vi "Previous Song.vi"(0 "reference in":refnum<class "MusicPlayer.lvclass">, 11 "Error In":errorcluster) -> (4 "reference out":refnum<class "MusicPlayer.lvclass">, 15 "Error Out":errorcluster)   [LabVIEW 2022 SP3, in "MusicPlayer.lvclass"]
uses:
  MusicPlayer.lvclass
  MusicPlayer.lvclass/MusicPlayer.ctl
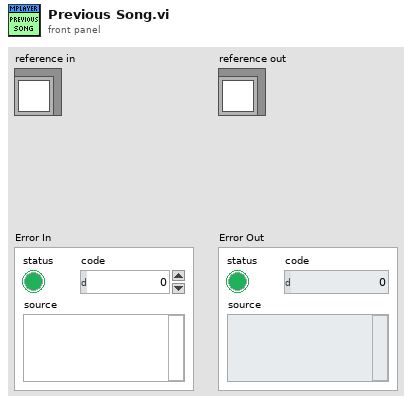
[diagram p1: front panel]
types:
  T1 = typedef "MusicPlayer.lvclass/ObjectAttributes.ctl" = cluster{"MediaPlayer":refnum<k7>, "Playlist":path[], "Index":u32}
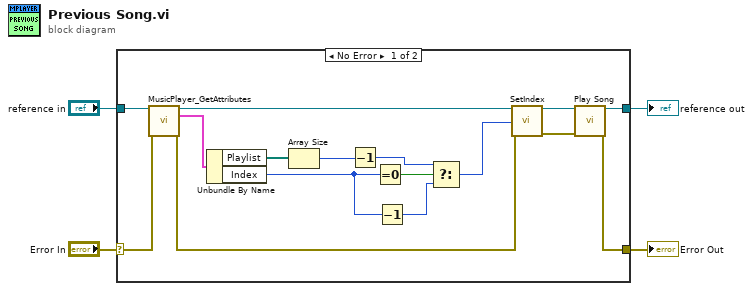
[diagram p0: block diagram]
diagram:
  n1 = case shown="No Error" "Error In" {
    selector: "Error In" -> [w20 w22]
    tunnel: [w8 w22] -> w3
    tunnel: [w6 w21] -> w1
    tunnel: "reference in" -> [w17 w21]
    frame No Error {
      n2 = call "MusicPlayer_GetAttributes.vi"("reference in"=w17, "error in (no error)"=w20) -> ("reference out"=w9:refnum<class "MusicPlayer.lvclass">, "Data"=w19:T1, "error out"=w18:errorcluster)  [unwired: 10 in, 1 out]
      n3 = Unbundle By Name(w19) -> ("Playlist"=w16:path[], "Index"=w12:u32)
      n4 = Array Size(array=w16) -> (size(s)=w14:i32)
      n5 = Decrement(x=w14) -> (x-1=w13:i32)
      n6 = Equal To 0?(x=w12) -> (x = 0?=w15:bool)
      n7 = Decrement(x=w12) -> (x-1=w11:u32)
      n8 = Select(t=w13, s=w15, f=w11) -> (s? t:f=w5:u32)
      n9 = call "SetIndex.vi"("reference in"=w9, "Index"=w5, "Error In"=w18) -> ("reference out"=w7:refnum<class "MusicPlayer.lvclass">, "Error Out"=w10:errorcluster)  [unwired: 11 in]
      n10 = call-dynamic "Play Song.vi"("reference in"=w7, "Error In"=w10) -> ("reference out"=w6:refnum<class "MusicPlayer.lvclass">, "Error Out"=w8:errorcluster)  [unwired: 12 in]
    }
    frame Error {
    }
  }
  "Error Out" <- w3
  "reference out" <- w1
